vi "init.vi"(8 "error in (no error)":errorcluster, 11 "MXN ACTOR in":refnum<class "MXN ACTOR.lvclass">) -> (0 "error out":errorcluster, 3 "MXN ACTOR out":refnum<class "MXN ACTOR.lvclass">)   [LabVIEW 2019, in "MXN ACTOR.lvlib" / "MXN ACTOR.lvclass"]
uses:
  MXN ACTOR.lvclass
  MXN ACTOR.lvclass/MXN ACTOR.ctl
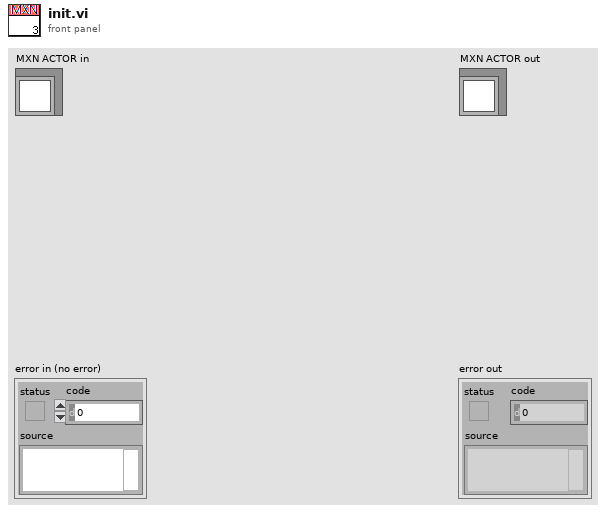
[diagram p1: front panel]
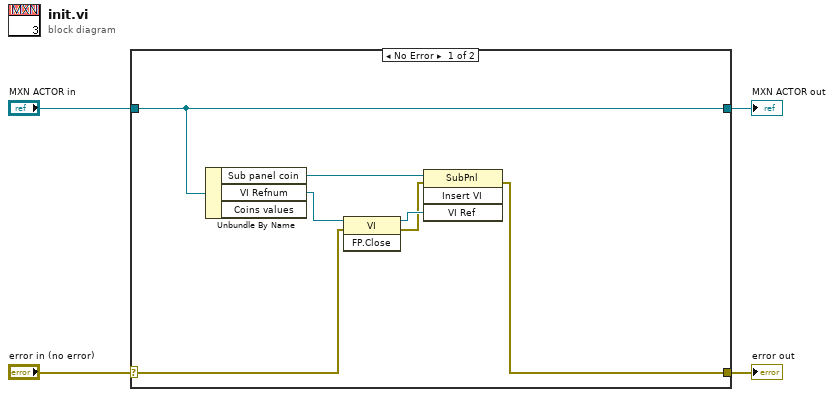
[diagram p0: block diagram]
diagram:
  n1 = case shown="No Error" "error in (no error)" {
    selector: "error in (no error)" -> [w7 w13]
    tunnel: [w6 w13] -> w3
    tunnel: [w5 w12] -> w1
    tunnel: "MXN ACTOR in" -> [w5 w12]
    frame No Error {
      n2 = Unbundle By Name(w5) -> ("Sub panel coin"=w9:refnum<vi>, "VI Refnum"=w10:refnum<vi>)  [unwired: 1 out]
      n3 = invoke class="VI" method="FP.Close"(reference=w10, error in=w7) -> (reference out=w11:refnum<vi>, error out=w8:errorcluster)  [unwired: 1 in, 1 out]
      n4 = invoke class="SubPnl" method="Insert VI"(reference=w9, error in=w8, "VI Ref"=w11) -> (error out=w6:errorcluster)  [unwired: 1 in, 3 out]
    }
    frame Error {
    }
  }
  "error out" <- w3
  "MXN ACTOR out" <- w1
